vi "GetTimerStatus.vi"(8 "error in (no error)":errorcluster, 10 "Name":string, 11 "TimerEngine in":refnum<class "TimerEngine.lvclass">) -> (0 "error out":errorcluster, 1 "Start?":bool, 2 "TimePeroid(ms)":i64, 3 "TimerEngine out":refnum<class "TimerEngine.lvclass">, 4 "EclipsedTime(ms)":i64, 5 "Exist?":bool)   [LabVIEW 2017, in "TimerEngine.lvlib" / "TimerEngine.lvclass"]
uses:
  TimerEngine.lvclass
  TimerEngine.lvclass/TimerEngine.ctl
  _TimerClass/Timer.lvclass
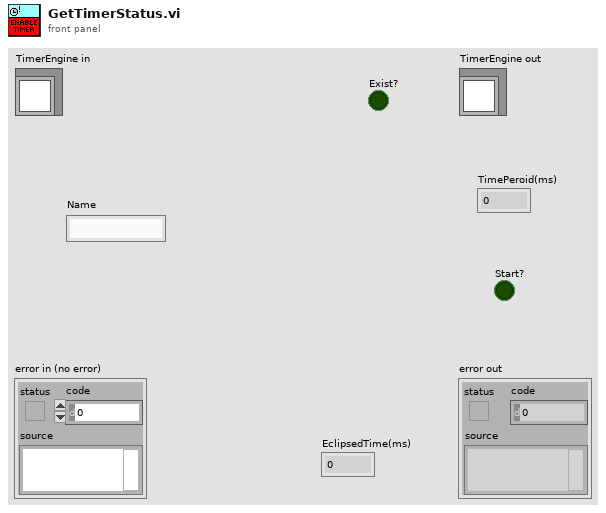
[diagram p1: front panel]
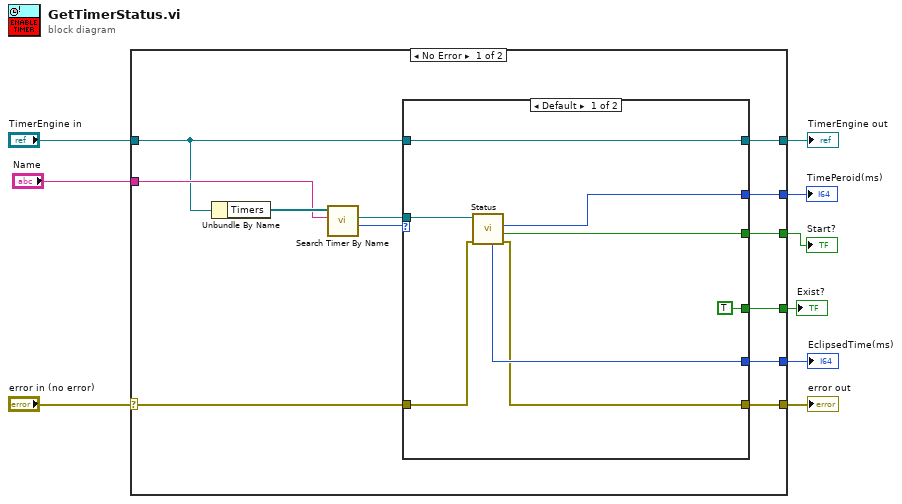
[diagram p0: block diagram]
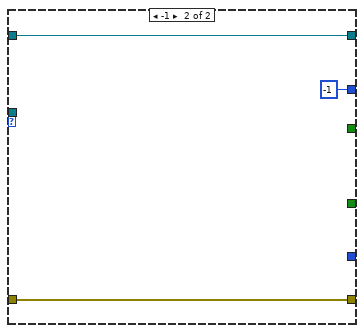
[diagram p2: hidden frame]
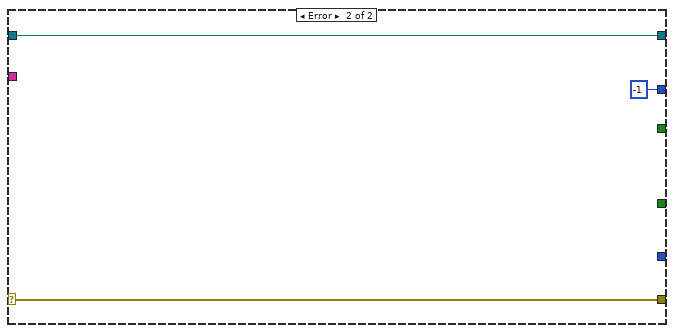
[diagram p3: hidden frame]
diagram:
  n1 = case shown="No Error" "error in (no error)" {
    selector: "error in (no error)" -> [w17 w35]
    tunnel: [w16 w35] -> w8
    tunnel: [w15 w34] -> w6
    tunnel: "TimerEngine in" -> [w14 w34]
    tunnel: "Name" -> [w20 _]
    tunnel: [w13 _] -> w4
    tunnel: [w12 i64 -1 ("TimePeroid(ms)")] -> w3
    tunnel: [w11 _] -> w2
    tunnel: [w10 _] -> w1
    frame No Error {
      n2 = Unbundle By Name(w14) -> ("Timers"=w21:refnum<class "Timer.lvclass">[])
      n3 = call "Search Timer By Name.vi"("Name"=w20, "Array"=w21) -> ("index of element"=w19:i32, "element"=w18:refnum<class "Timer.lvclass">)  [unwired: 6 in, 2 out]
      n4 = case shown="Default" w19 {
        tunnel: w18 -> [w27 _]
        tunnel: w17 -> [w23 w32]
        tunnel: [w22 w32] -> w16
        tunnel: [w29 w31] -> w15
        tunnel: w14 -> [w29 w31]
        tunnel: [TRUE _] -> w13
        tunnel: [w26 i64 -1 ("TimePeroid(ms)")] -> w12
        tunnel: [w25 _] -> w11
        tunnel: [w24 _] -> w10
        frame Default {
          n5 = call "Status.vi"("error in (no error)"=w23, "Timer in"=w27) -> ("error out"=w22:errorcluster, "Start?"=w25:bool, "TimePeroid(ms)"=w26:i64, "EclipsedTime(ms)"=w24:i64)  [unwired: 5 in, 1 out]
        }
        frame -1 {
        }
      }
    }
    frame Error {
    }
  }
  "error out" <- w8
  "TimerEngine out" <- w6
  "Exist?" <- w4
  "TimePeroid(ms)" <- w3
  "Start?" <- w2
  "EclipsedTime(ms)" <- w1
